vi "Stop (SubVI).vi"(11 "VISA Refnum in":refnum<visa-resource-name>) -> ()   [LabVIEW 2021]
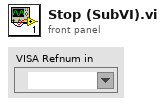
[diagram p1: front panel]
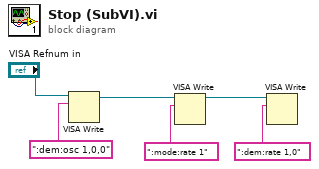
[diagram p0: block diagram]
diagram:
  n1 = VISA Write(VISA resource name="VISA Refnum in", write buffer=":dem:osc 1,0,0") -> (VISA resource name out=w3:refnum<visa-resource-name>)  [unwired: 1 in, 2 out]
  n2 = VISA Write(VISA resource name=w3, write buffer=":mode:rate 1") -> (VISA resource name out=w5:refnum<visa-resource-name>)  [unwired: 1 in, 2 out]
  n3 = VISA Write(VISA resource name=w5, write buffer=":dem:rate 1,0") -> ()  [unwired: 1 in, 3 out]
